vi "Inverse Kinematics (Point).vi"(5 "max steps":i32=100, 7 "mask":dbl[](array[numeric]), 8 "error in (no error)":errorcluster, 9 "current joint positions":dbl[](array[numeric]), 10 "end effector transform":T1, 11 "serial arm in":refnum<class "NI_Robotics_Serial Robot Arm.lvclass">) -> (0 "error out":errorcluster, 1 "steps taken":i32, 2 "joint positions":dbl[](array[numeric]), 3 "serial arm out":refnum<class "NI_Robotics_Serial Robot Arm.lvclass">)   [LabVIEW 2017, in "NI_Kinematics.lvlib"]
doc: "Computes the joint angles of a robotic arm given the location of the end effector relative to the arm base. Wire data to the <B>end effector transform</B> input to determine the polymorphic instance to use or manually select the instance.\n\n<B>.m file:</B> ikine"
uses:
  <vilib>/robotics/Kinematics/NI_Kinematics.lvlib
  <vilib>/robotics/Kinematics/Robot/NI_Robotics_Serial Robot Arm.lvclass
  <vilib>/Analysis/Matrix/Datatypes/RealMatrix.ctl
  <vilib>/Analysis/_algsub.llb/Real Vector Norm.vi
  <vilib>/robotics/Kinematics/Transform2ToDiff.vi
  <vilib>/Analysis/7linalg.llb/Solve Linear Equations (single right hand).vi
  <vilib>/Analysis/baseanly.llb/Solve Linear Equations By Cholesky.vi
  <vilib>/Analysis/baseanly.llb/Real Matrix to Compact Array.vi
  <vilib>/Analysis/baseanly.llb/Real Compact Tri-Matrix Linear Eqs.vi
  <vilib>/Analysis/7linalg.llb/Solve Linear Eqs (General).vi
  <vilib>/Analysis/7linalg.llb/Solve Linear Eqs (Gen, single right hand).vi
  <vilib>/Analysis/coordinate.llb/Cross Product.vi
  <vilib>/Analysis/NI_AALPro.lvlib
  <vilib>/robotics/Utilities/NI_Robotics Utilities.lvlib
  <vilib>/Analysis/Matrix/NI_Matrix.lvlib
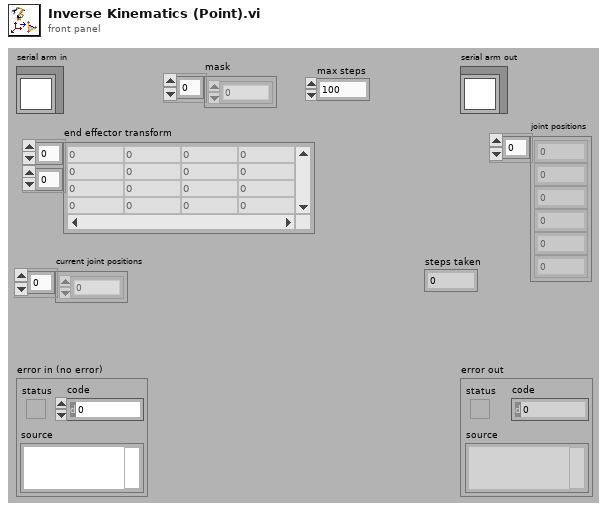
[diagram p1: front panel]
types:
  T1 = typedef "NI_Matrix.lvlib/RealMatrix.ctl" = dbl[][]
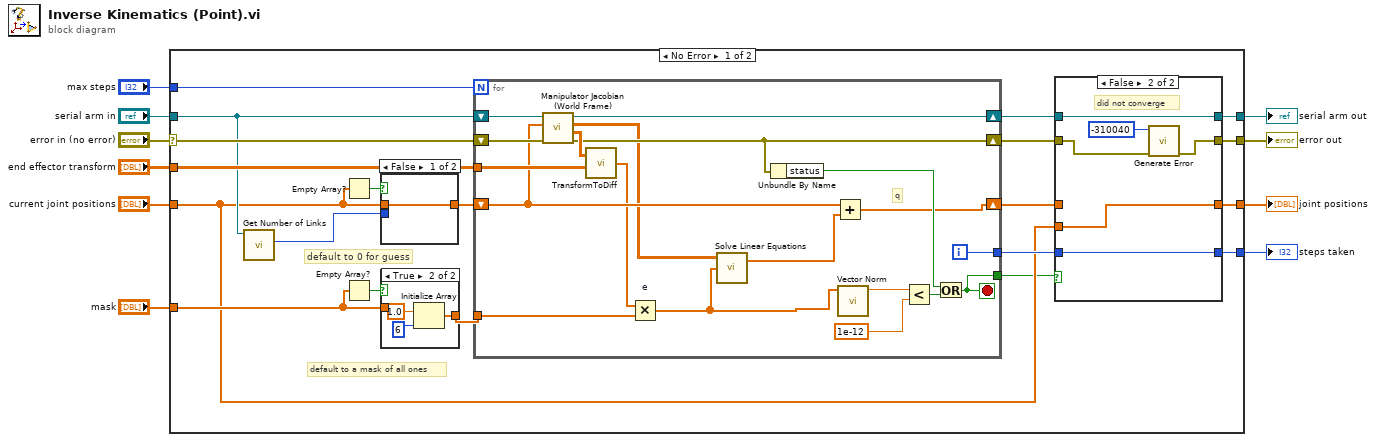
[diagram p0: block diagram]
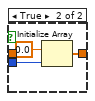
[diagram p3: hidden frame]
diagram:
  n1 = case shown="No Error" "error in (no error)" {
    selector: "error in (no error)" -> [w26 w70]
    tunnel: [w15 w70] -> w9
    tunnel: [w14 w69] -> w7
    tunnel: "serial arm in" -> [w22 w69]
    tunnel: "mask" -> [w29 _]
    tunnel: "current joint positions" -> [w12 w68]
    tunnel: "end effector transform" -> [w27 _]
    tunnel: [w17 w68] -> w3
    tunnel: [w19 _] -> w2
    tunnel: "max steps" -> [w21 _]
    frame No Error {
      # "default to a mask of all ones"
      # "default to 0 for guess"
      n2 = call <vilib>:"Get Number of Links.vi"("serial arm in"=w22) -> ("number of links"=w23:i32)  [unwired: 8 in, 2 out]
      n3 = Empty Array?(array=w12) -> (empty?=w25:bool)
      n4 = Empty Array?(array=w29) -> (empty?=w30:bool)
      n5 = case shown="False" w25 {
        tunnel: w12 -> [w41 _]
        tunnel: [w41 w42] -> w24
        tunnel: w23 -> [_ w43]
        frame False {
        }
        frame True {
          n6 = Initialize Array(0.0 ("element"), w43) -> (w42:dbl[])
        }
      }
      n7 = case shown="True" w30 {
        tunnel: w29 -> [w64 _]
        tunnel: [w64 w66] -> w28
        frame False {
        }
        frame True {
          n8 = Initialize Array(1.0 ("element"), 6 ("dimension size")) -> (w66:dbl[])
        }
      }
      n9 = for {
        N: w21 -> [_]
        tunnel: w28 -> [w63]
        shift-right: [w46] -> w18
        shift-left: w24 -> [w53]
        tunnel: w27 -> [w60]
        shift-right: [w56] -> w16
        shift-left: w26 -> [w58]
        shift-right: [w62] -> w13
        shift-left: w22 -> [w59]
        tunnel: [w51] -> w20
        tunnel: [w50] -> w11
        i -> [w51]
        stop <- w50 stop-if-true
        # "q"
        n10 = call <vilib>:"Manipulator Jacobian (World Frame).vi"("error in (no error)"=w58, "joint positions"=w53, "serial arm in"=w59) -> ("error out"=w56:errorcluster, "forward kinematics"=w57:T1, "jacobian"=w49:T1, "serial arm out"=w62:refnum<class "NI_Robotics_Serial Robot Arm.lvclass">)  [unwired: 5 out]
        n11 = call-poly <vilib>:"TransformToDiff.vi"("End Transform"=w60, "Start Transform"=w57) -> ("Differential"=w52:dbl[])
        n12 = Multiply "e"(x=w52, y=w63) -> (x*y=w47:dbl[])
        n13 = call-poly <vilib>:"Solve Linear Equations.vi"("Known Vector"=w47, "Input Matrix"=w49) -> ("Solution Vector"=w48:dbl[])  [unwired: 1 in, 1 out]
        n14 = Unbundle By Name(w56) -> ("status"=w54:bool)
        n15 = Add ("Add.vi")(x=w53, y=w48) -> (x+y=w46:dbl[])
        n16 = call-poly <vilib>:"Vector Norm.vi"("Input Vector"=w47) -> ("norm"=w45:dbl)  [unwired: 2 in, 8 out]
        n17 = Less?(x=w45, y=1e-12 ("element")) -> (x < y?=w55:bool)
        n18 = Or(x=w54, y=w55) -> (x .or. y?=w50:bool)
      }
      n19 = case shown="False" w11 {
        tunnel: w20 -> [w31 w40]
        tunnel: [w31 w40] -> w19
        tunnel: w18 -> [w32 _]
        tunnel: [w32 w35] -> w17
        tunnel: w16 -> [w33 w37]
        tunnel: [w33 w36] -> w15
        tunnel: [w34 w39] -> w14
        tunnel: w13 -> [w34 w39]
        tunnel: w12 -> [_ w35]
        frame True {
        }
        frame False {
          # "did not converge"
          n20 = call <vilib>:"Generate Error.vi"("error in (no error)"=w37, "code"=-310040) -> ("error out"=w36:errorcluster)  [unwired: 9 in]
        }
      }
    }
    frame Error {
    }
  }
  "error out" <- w9
  "serial arm out" <- w7
  "joint positions" <- w3
  "steps taken" <- w2
